vi "Acquire_Waveform_example.vi"() -> ()   [LabVIEW 2011]
doc: "Demonstrates how to set up an oscilloscope automatically. You can configure this VI to acquire a waveform from a single channel by following the following steps:\n\n1. Specify a valid VISA resource to use. \n2. Specify a channel. \n3. Specify a time-out value for reading a waveform.\n4. Run this VI. The <B>Waveform Graph</B> displays the waveform you acquire."
uses:
  <instrlib>/Tektronix 7000 Series/Public/Data/Read (Single Waveform).vi
  <instrlib>/Tektronix 7000 Series/Tektronix 7000 Series.lvlib
panel:
  in  "Maximum Time (10000 ms)":u32=10000
  in  "Probe Attenuation (10)":dbl=10.0
  in  "Channel (0: Channel 1)":u16(ring) format="%#_5f" items=["Channel 1", "Channel 2", "Channel 3", "Channel 4", "Math 1", "Math 2", "Math 3", "Math 4", "Reference 1", "Reference 2", "Reference 3", "Reference 4"]
  in  "VISA Resource Name":refnum<visa-resource-name>
  out "Waveform Graph":waveform(dbl)(graph)
  # "(c) 2006. National Instruments Corporation. ALL RIGHTS RESERVED."
  # "(c) 2006 - 2011 National Instruments Corporation.  ALL RIGHTS RESERVED."
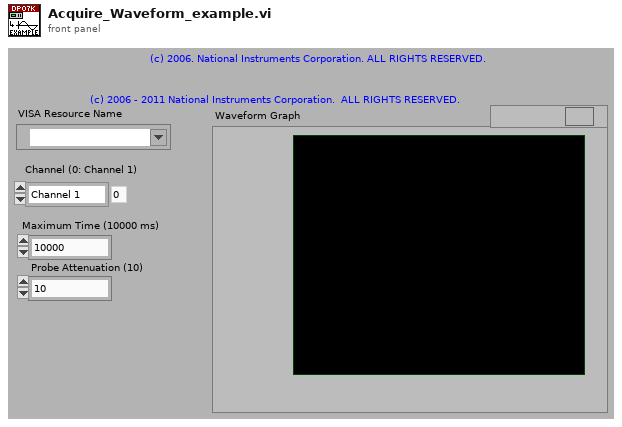
[diagram p1: front panel]
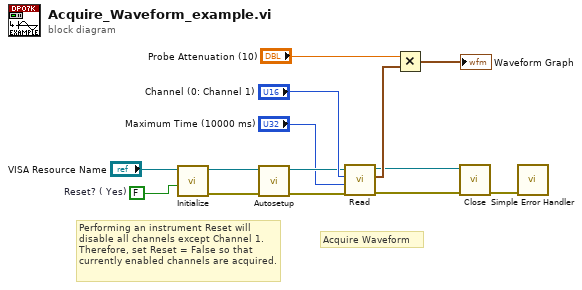
[diagram p0: block diagram]
diagram:
  w1 = FALSE  # Reset? ( Yes)
  # "Performing an instrument Reset will disable all channels except Channel 1. Therefore, set Reset = False so that currently enabled channels are acquired."
  # "Acquire Waveform"
  n1 = call <instrlib>:"Initialize.vi"("Reset? ( Yes)"=w1, "VISA resource name"="VISA Resource Name") -> ("error out"=w5:errorcluster, "VISA resource name out"=w6:refnum<visa-resource-name>)  [unwired: 8 in]
  n2 = call <instrlib>:"Autosetup.vi"("error in (no error)"=w5, "VISA resource name"=w6) -> ("error out"=w3:errorcluster, "VISA resource name out"=w4:refnum<visa-resource-name>)  [unwired: 8 in]
  n3 = call-poly <instrlib>:"Read.vi"("error in (no error)"=w3, "Maximum Time (10000 ms)"="Maximum Time (10000 ms)", "Channel (0: Channel 1)"="Channel (0: Channel 1)", "VISA resource name"=w4) -> ("error out"=w8:errorcluster, "Waveform Data"=w10:waveform(dbl), "VISA resource name out"=w9:refnum<visa-resource-name>)  [unwired: 5 in]
  n4 = Multiply(x="Probe Attenuation (10)", y=w10) -> (x*y=→"Waveform Graph":waveform(dbl))
  n5 = call <instrlib>:"Close.vi"("error in (no error)"=w8, "VISA resource name"=w9) -> ("error out"=w14:errorcluster)  [unwired: 9 in]
  n6 = call <vilib>:"Simple Error Handler.vi"("error in (no error)"=w14) -> ()  [unwired: 4 in, 5 out]
